vi "Flush Buffer.vi"(8 "error in":errorcluster, 11 "Tasks In":refnum<k21>) -> (0 "error out":errorcluster, 3 "Tasks Out":refnum<k21>)   [LabVIEW 2018]
doc: "Reads all available samples on all input DAQmx Tasks. Use this to periodically empty the buffer to compensate for clock drift without the hassles of synchronization."
uses:
  <vilib>/DAQmx/read.llb/DAQmx Read (Analog 2D DBL NChan NSamp).vi
  <vilib>/DAQmx/miscellaneous.llb/DAQmx Fill In Error Info.vi
  <resource>/objmgr/daqmx.rc
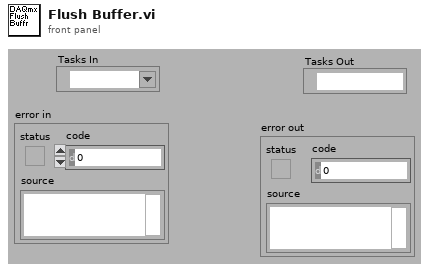
[diagram p1: front panel]
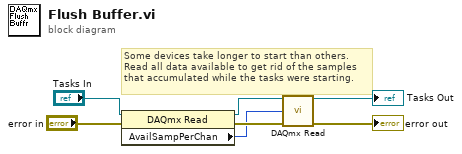
[diagram p0: block diagram]
diagram:
  # "Some devices take longer to start than others.\nRead all data available to get rid of the samples\nthat accumulated while the tasks were starting."
  n1 = property class="DAQmx Read"(reference="Tasks In", error in="error in") -> (reference out=w2:refnum<k21>, error out=w3:errorcluster, "AvailSampPerChan"=w1:u32)
  n2 = call-poly <vilib>:"DAQmx Read.vi"("task/channels in"=w2, "number of samples per channel"=w1, "error in"=w3) -> ("task out"=→"Tasks Out":refnum<k21>, "error out"=→"error out":errorcluster)  [unwired: 10 in, 1 out]
